vi "Heater Monitor.vi"() -> ()   [LabVIEW 2017]
uses:
  <vilib>/Utility/error.llb/Clear Errors.vi
  <instrlib>/tio-labview/TIO Library/Data Stream/TIO Data Stream Parse Description.vi
panel:
  in  "Voltage Max":dbl[unit] format="%#_4g"
  in  "Voltage Full Scale":dbl[unit] format="%#_4g"
  in  "Voltage":dbl[unit] format="%#_4g"
  in  "Manual":bool
  in  "Freq":dbl[unit] format="%#_4g"
  in  "Autostart":bool
  in  "Ki":dbl format="%#_4g"
  in  "Kp":dbl format="%#_4g"
  out "Resistance Measured":dbl[unit] format="%#_4g"
  in  "Save":bool
  in  "Calibrate R0":bool
  in  "Load":dbl[unit] format="%#_4g"
  in  "Heater Enable":bool
  out "Power Output":dbl[unit] format="%#_4f"
  in  "Power Max":dbl[unit] format="%#_4f"
  out "Temperature Measured":dbl[unit] format="%#_4g"
  in  "Temperature Set":dbl[unit] format="%#_4g"
  out "Kill":bool=TRUE
  in  "URL":refnum<visa-resource-name>="tcp://localhost"
  out "ID":string="Twinleaf VM4 R4"
  in  "Quit":bool
  in  "Duration":dbl[unit]=1000.0
  in  "Reset":bool
  out "Temperature":cluster{dbl, dbl, dbl[]}(graph)={407.109653, 0.002, []}
  # "Heater Monitor"
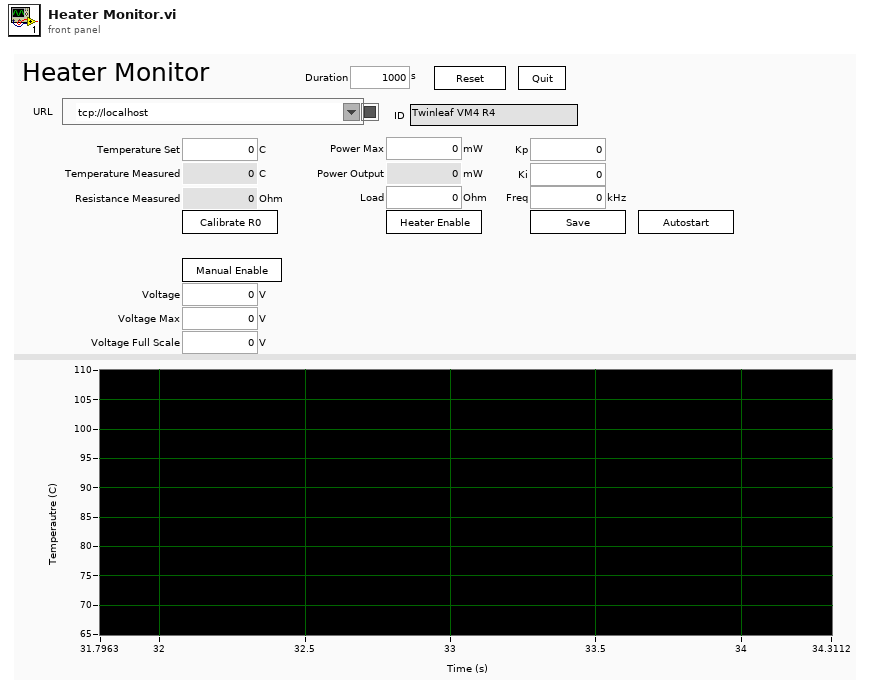
[diagram p1: front panel]
types:
  T1 = cluster{"Type":enum16{"TCP", "Serial"}, "Serial":refnum<visa-resource-name>, "TCP":refnum<k5>, "Timeout":u32}
  T2 = cluster{"Stream Description":cluster{"Stream ID":u16, "Data Type":u8, "Channels":u8, "Restart ID":u16, "Start timestamp (s)":dbl, "Sample counter":u64, "Period (s)":dbl, "Flags":u8, "Timestamp type":u8, "Name":string, "Last sample number":u64, "Last Restart ID":u16, "Version":u16, "Sample Size":u16}, "Sample #":u32, "Raw Data":string}
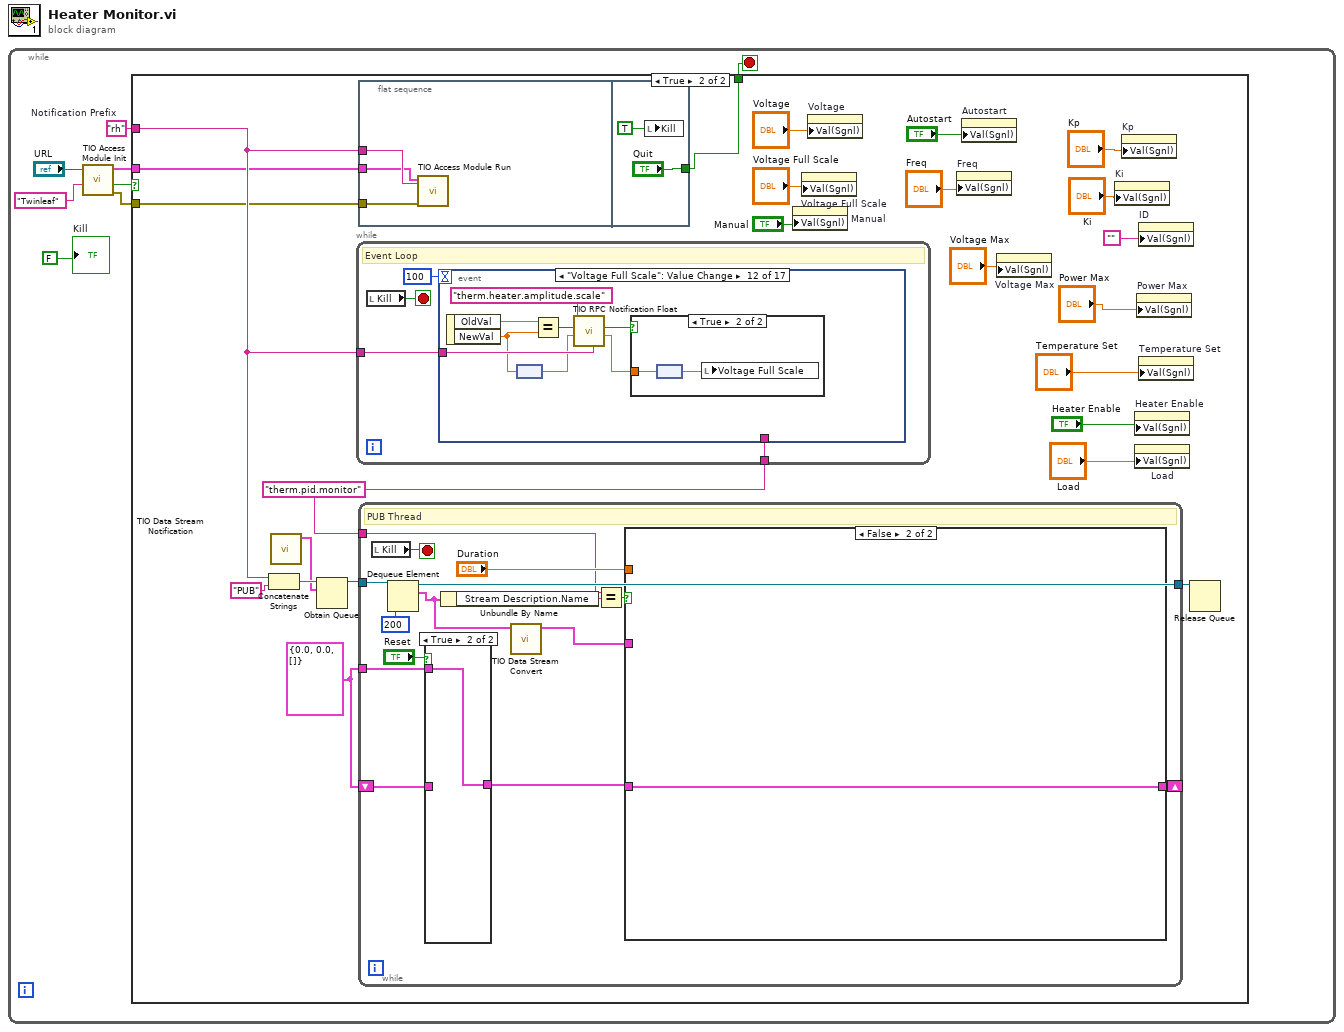
[diagram p0: block diagram]
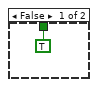
[diagram p2: hidden frame]
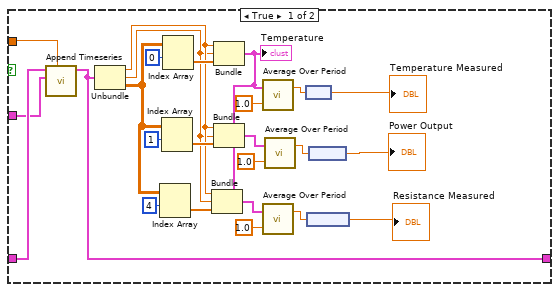
[diagram p4: hidden frame]
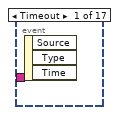
[diagram p5: hidden frame]
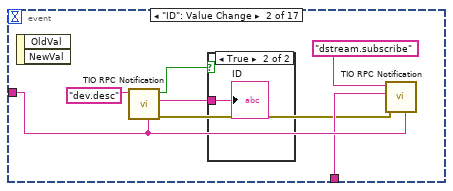
[diagram p6: hidden frame]
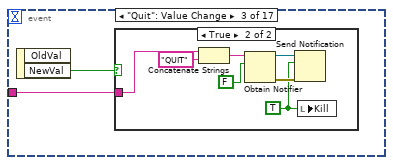
[diagram p8: hidden frame]
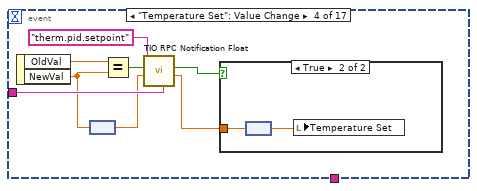
[diagram p10: hidden frame]
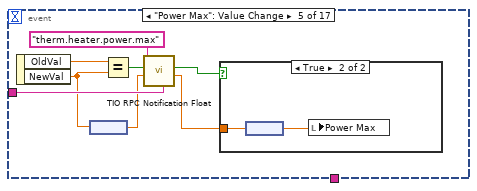
[diagram p12: hidden frame]
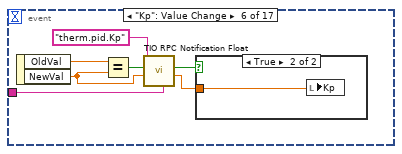
[diagram p14: hidden frame]
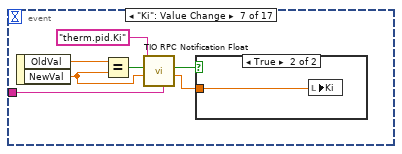
[diagram p16: hidden frame]
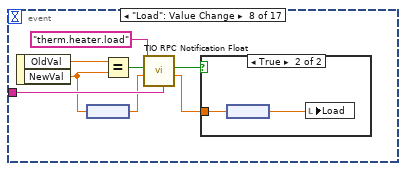
[diagram p18: hidden frame]
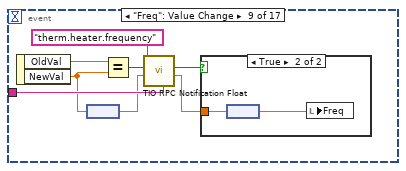
[diagram p20: hidden frame]
diagram:
  n1 = while {
    stop <- w1 stop-if-true
    w8 = "rh"  # Notification Prefix
    n2 = call <instrlib>:"TIO Access Module Init.vi"("ID"="Twinleaf", "URL"="URL") -> ("error out"=w5:errorcluster, "Connected"=w3:bool, "TS Connection"=w4:T1)  [unwired: 7 in]
    n3 = case shown="True" w3 {
      tunnel: w8 -> [_ w33]
      tunnel: w5 -> [_ w32]
      tunnel: w4 -> [_ w31]
      tunnel: [TRUE ("Quit") w14] -> w1
      frame False {
      }
      frame True {
        w15 = "therm.pid.monitor" ("Topic")
        w25 = cluster{dbl, dbl, dbl[][]} {0.0, 0.0, []} ("Waveform Timeseries")
        n4 = Concatenate Strings(w33, "PUB" ("name (unnamed)")) -> (w29:string)
        n5 = call <instrlib>:"TIO Data Stream Notification.vi"() -> ("Data Stream Notification"=w24:T2)  [unwired: 11 in]
        n6 = Obtain Queue(name (unnamed)=w29, element data type=w24) -> (queue out=w27:refnum<queue>)  [unwired: 3 in, 2 out]
        n7 = while {
          tunnel: w33 -> [w78]
          tunnel: w15 -> [w77]
          stop <- w80 stop-if-true
          # "Event Loop"
          n8 = local read "Kill"() -> (w80:bool)
          n9 = event shown="[11] \"Voltage Full Scale\": Value Change" {
            selector: _ -> [_ _ _ _ _ _ _ _ _ _ _ _ _ _ _ _ _]
            dyn-events: _ -> [_ _ _ _ _ _ _ _ _ _ _ _ _ _ _ _ _]
            timeout: 100 -> [_ _ _ _ _ _ _ _ _ _ _ _ _ _ _ _ _]
            tunnel: w78 -> [_ w83 w89 w105 w115 w124 w132 w141 w151 w161 w171 w181 w189 w199 w209 w215 w217]
            tunnel: w77 -> [_ w82 _ _ _ _ _ _ _ _ _ _ _ _ _ _ _]
            event Timeout {
              n10 = event-data() -> ()  [unwired: 1 in, 3 out]
            }
            event "ID": Value Change {
              n11 = event-data() -> ()  [unwired: 1 in, 2 out]
              n12 = call <instrlib>:"TIO RPC Notification.vi"("Notification Prefix"=w83, "Topic"="dev.desc") -> ("error out"=w81:errorcluster, "REP"=w86:string, "Response"=w85:bool)  [unwired: 6 in]
              n13 = case shown="True" w85 {
                tunnel: w86 -> [_ w88]
                frame False {
                }
                frame True {
                  "ID" <- w88
                }
              }
              n14 = call <instrlib>:"TIO RPC Notification.vi"("Notification Prefix"=w83, "error in (no error)"=w81, "Payload"=w82, "Topic"="dstream.subscribe") -> ()  [unwired: 4 in, 3 out]
            }
            event "Quit": Value Change {
              n15 = event-data() -> ("NewVal"=w90:bool)  [unwired: 1 in, 1 out]
              n16 = case shown="True" w90 {
                tunnel: w89 -> [_ w91]
                frame False {
                }
                frame True {
                  w92 = TRUE ("Kill")
                  n17 = Concatenate Strings(w91, "QUIT" ("name (unnamed)")) -> (w97:string)
                  n18 = Obtain Notifier(name (unnamed)=w97, notification data type=FALSE ("Connected")) -> (notifier out=w94:refnum<notifier>, error out=w95:errorcluster)  [unwired: 2 in, 1 out]
                  n19 = Send Notification(notification=w92, notifier=w94, error in (no error)=w95) -> ()  [unwired: 2 out]
                  n20 = local write "Kill"(w92) -> ()
                }
              }
            }
            event "Temperature Set": Value Change {
              n21 = event-data() -> ("OldVal"=w104:dbl[unit], "NewVal"=w98:dbl[unit])  [unwired: 1 in]
              n22 = node(w98) -> (w102:dbl)
              n23 = Equal?(x=w104, y=w98) -> (x = y?=w103:bool)
              n24 = call <instrlib>:"TIO RPC Notification Float.vi"("Notification"=w105, "Set value"=w102, "Read"=w103, "String"="therm.pid.setpoint") -> ("Get value (default if error)"=w100:sgl, "Response"=w101:bool)  [unwired: 4 in, 1 out]
              n25 = case shown="True" w101 {
                tunnel: w100 -> [_ w107]
                frame False {
                }
                frame True {
                  n26 = node(w107) -> (w106:sgl[unit])
                  n27 = local write "Temperature Set"(w106) -> ()
                }
              }
            }
            event "Power Max": Value Change {
              n28 = event-data() -> ("OldVal"=w114:dbl[unit], "NewVal"=w108:dbl[unit])  [unwired: 1 in]
              n29 = node(w108) -> (w112:dbl)
              n30 = Equal?(x=w114, y=w108) -> (x = y?=w113:bool)
              n31 = call <instrlib>:"TIO RPC Notification Float.vi"("Notification"=w115, "Set value"=w112, "Read"=w113, "String"="therm.heater.power.max") -> ("Get value (default if error)"=w110:sgl, "Response"=w111:bool)  [unwired: 4 in, 1 out]
              n32 = case shown="True" w111 {
                tunnel: w110 -> [_ w117]
                frame False {
                }
                frame True {
                  n33 = node(w117) -> (w116:sgl[unit])
                  n34 = local write "Power Max"(w116) -> ()
                }
              }
            }
            event "Kp": Value Change {
              n35 = event-data() -> ("OldVal"=w123:dbl, "NewVal"=w118:dbl)  [unwired: 1 in]
              n36 = Equal?(x=w123, y=w118) -> (x = y?=w122:bool)
              n37 = call <instrlib>:"TIO RPC Notification Float.vi"("Notification"=w124, "Set value"=w118, "Read"=w122, "String"="therm.pid.Kp") -> ("Get value (default if error)"=w120:sgl, "Response"=w121:bool)  [unwired: 4 in, 1 out]
              n38 = case shown="True" w121 {
                tunnel: w120 -> [_ w125]
                frame False {
                }
                frame True {
                  n39 = local write "Kp"(w125) -> ()
                }
              }
            }
            event "Ki": Value Change {
              n40 = event-data() -> ("OldVal"=w131:dbl, "NewVal"=w126:dbl)  [unwired: 1 in]
              n41 = Equal?(x=w131, y=w126) -> (x = y?=w130:bool)
              n42 = call <instrlib>:"TIO RPC Notification Float.vi"("Notification"=w132, "Set value"=w126, "Read"=w130, "String"="therm.pid.Ki") -> ("Get value (default if error)"=w128:sgl, "Response"=w129:bool)  [unwired: 4 in, 1 out]
              n43 = case shown="True" w129 {
                tunnel: w128 -> [_ w133]
                frame False {
                }
                frame True {
                  n44 = local write "Ki"(w133) -> ()
                }
              }
            }
            event "Load": Value Change {
              n45 = event-data() -> ("OldVal"=w140:dbl[unit], "NewVal"=w134:dbl[unit])  [unwired: 1 in]
              n46 = node(w134) -> (w138:dbl)
              n47 = Equal?(x=w140, y=w134) -> (x = y?=w139:bool)
              n48 = call <instrlib>:"TIO RPC Notification Float.vi"("Notification"=w141, "Set value"=w138, "Read"=w139, "String"="therm.heater.load") -> ("Get value (default if error)"=w136:sgl, "Response"=w137:bool)  [unwired: 4 in, 1 out]
              n49 = case shown="True" w137 {
                tunnel: w136 -> [_ w143]
                frame False {
                }
                frame True {
                  n50 = node(w143) -> (w142:sgl[unit])
                  n51 = local write "Load"(w142) -> ()
                }
              }
            }
            event "Freq": Value Change {
              n52 = event-data() -> ("OldVal"=w150:dbl[unit], "NewVal"=w144:dbl[unit])  [unwired: 1 in]
              n53 = node(w144) -> (w148:dbl)
              n54 = Equal?(x=w150, y=w144) -> (x = y?=w149:bool)
              n55 = call <instrlib>:"TIO RPC Notification Float.vi"("Notification"=w151, "Set value"=w148, "Read"=w149, "String"="therm.heater.frequency") -> ("Get value (default if error)"=w146:sgl, "Response"=w147:bool)  [unwired: 4 in, 1 out]
              n56 = case shown="True" w147 {
                tunnel: w146 -> [_ w153]
                frame False {
                }
                frame True {
                  n57 = node(w153) -> (w152:sgl[unit])
                  n58 = local write "Freq"(w152) -> ()
                }
              }
            }
            event "Voltage": Value Change {
              n59 = event-data() -> ("OldVal"=w160:dbl[unit], "NewVal"=w154:dbl[unit])  [unwired: 1 in]
              n60 = node(w154) -> (w158:dbl)
              n61 = Equal?(x=w160, y=w154) -> (x = y?=w159:bool)
              n62 = call <instrlib>:"TIO RPC Notification Float.vi"("Notification"=w161, "Set value"=w158, "Read"=w159, "String"="therm.heater.amplitude") -> ("Get value (default if error)"=w156:sgl, "Response"=w157:bool)  [unwired: 4 in, 1 out]
              n63 = case shown="True" w157 {
                tunnel: w156 -> [_ w163]
                frame False {
                }
                frame True {
                  n64 = node(w163) -> (w162:sgl[unit])
                  n65 = local write "Voltage"(w162) -> ()
                }
              }
            }
            event "Voltage Max": Value Change {
              n66 = event-data() -> ("OldVal"=w170:dbl[unit], "NewVal"=w164:dbl[unit])  [unwired: 1 in]
              n67 = node(w164) -> (w168:dbl)
              n68 = Equal?(x=w170, y=w164) -> (x = y?=w169:bool)
              n69 = call <instrlib>:"TIO RPC Notification Float.vi"("Notification"=w171, "Set value"=w168, "Read"=w169, "String"="therm.heater.amplitude.max") -> ("Get value (default if error)"=w166:sgl, "Response"=w167:bool)  [unwired: 4 in, 1 out]
              n70 = case shown="True" w167 {
                tunnel: w166 -> [_ w173]
                frame False {
                }
                frame True {
                  n71 = node(w173) -> (w172:sgl[unit])
                  n72 = local write "Voltage Max"(w172) -> ()
                }
              }
            }
            event "Voltage Full Scale": Value Change {
              n73 = event-data() -> ("OldVal"=w180:dbl[unit], "NewVal"=w174:dbl[unit])  [unwired: 1 in]
              n74 = node(w174) -> (w178:dbl)
              n75 = Equal?(x=w180, y=w174) -> (x = y?=w179:bool)
              n76 = call <instrlib>:"TIO RPC Notification Float.vi"("Notification"=w181, "Set value"=w178, "Read"=w179, "String"="therm.heater.amplitude.scale") -> ("Get value (default if error)"=w176:sgl, "Response"=w177:bool)  [unwired: 4 in, 1 out]
              n77 = case shown="True" w177 {
                tunnel: w176 -> [_ w183]
                frame False {
                }
                frame True {
                  n78 = node(w183) -> (w182:sgl[unit])
                  n79 = local write "Voltage Full Scale"(w182) -> ()
                }
              }
            }
            event "Heater Enable": Value Change {
              n80 = event-data() -> ("OldVal"=w191:bool, "NewVal"=w184:bool)  [unwired: 1 in]
              n81 = Equal?(x=w191, y=w184) -> (x = y?=w188:bool)
              n82 = Boolean To (0,1)(Boolean=w184) -> (0, 1=w190:i16)
              n83 = call <instrlib>:"TIO RPC Notification U8.vi"("Notification Prefix"=w189, "U8"=w190, "Read"=w188, "String"="therm.pid.enable") -> ("U8"=w185:u8, "Response"=w186:bool)  [unwired: 4 in, 1 out]
              n84 = case shown="True" w186 {
                tunnel: w185 -> [_ w193]
                frame False {
                }
                frame True {
                  n85 = Greater Than 0?(x=w193) -> (x > 0?=w192:bool)
                  n86 = local write "Heater Enable"(w192) -> ()
                }
              }
            }
            event "Autostart": Value Change {
              n87 = event-data() -> ("OldVal"=w201:bool, "NewVal"=w194:bool)  [unwired: 1 in]
              n88 = Equal?(x=w201, y=w194) -> (x = y?=w198:bool)
              n89 = Boolean To (0,1)(Boolean=w194) -> (0, 1=w200:i16)
              n90 = call <instrlib>:"TIO RPC Notification U8.vi"("Notification Prefix"=w199, "U8"=w200, "Read"=w198, "String"="autostart") -> ("U8"=w195:u8, "Response"=w196:bool)  [unwired: 4 in, 1 out]
              n91 = case shown="True" w196 {
                tunnel: w195 -> [_ w203]
                frame False {
                }
                frame True {
                  n92 = Greater Than 0?(x=w203) -> (x > 0?=w202:bool)
                  n93 = local write "Autostart"(w202) -> ()
                }
              }
            }
            event "Manual": Value Change {
              n94 = event-data() -> ("OldVal"=w211:bool, "NewVal"=w204:bool)  [unwired: 1 in]
              n95 = Equal?(x=w211, y=w204) -> (x = y?=w208:bool)
              n96 = Boolean To (0,1)(Boolean=w204) -> (0, 1=w210:i16)
              n97 = call <instrlib>:"TIO RPC Notification U8.vi"("Notification Prefix"=w209, "U8"=w210, "Read"=w208, "String"="therm.pid.manual") -> ("U8"=w205:u8, "Response"=w206:bool)  [unwired: 4 in, 1 out]
              n98 = case shown="True" w206 {
                tunnel: w205 -> [_ w213]
                frame False {
                }
                frame True {
                  n99 = Greater Than 0?(x=w213) -> (x > 0?=w212:bool)
                  n100 = local write "Manual"(w212) -> ()
                }
              }
            }
            event "Calibrate R0": Value Change {
              n101 = event-data() -> ()  [unwired: 1 in, 2 out]
              n102 = call <instrlib>:"TIO RPC Notification.vi"("Notification Prefix"=w215, "Topic"="therm.R0.capture" ("String")) -> ()  [unwired: 6 in, 3 out]
            }
            event "Save": Value Change {
              n103 = event-data() -> ()  [unwired: 1 in, 2 out]
              n104 = call <instrlib>:"TIO RPC Notification.vi"("Notification Prefix"=w217, "Topic"="conf.save" ("String")) -> ()  [unwired: 6 in, 3 out]
            }
          }
        }
        n105 = flat-sequence {
          tunnel: w33 -> [w220]
          tunnel: w32 -> [w219]
          tunnel: w31 -> [w218]
          tunnel: ["Quit"] -> _
          tunnel: ["Quit"] -> w14
          frame #0 {
            n106 = call <instrlib>:"TIO Access Module Run.vi"("Notification Prefix"=w220, "error in (no error)"=w219, "TS Connection"=w218) -> ()  [unwired: 9 in]
          }
          frame #1 {
            n107 = local write "Kill"(TRUE ("Kill")) -> ()
          }
        }
        n108 = while {
          tunnel: w27 -> [w46]
          shift-right: [w45] -> _
          shift-left: w25 -> [w43]
          tunnel: w25 -> [w42]
          tunnel: [w39] -> w26
          tunnel: w15 -> [w34]
          stop <- w47 stop-if-true
          # "PUB Thread"
          n109 = local read "Kill"() -> (w47:bool)
          n110 = Dequeue Element(queue=w46, timeout in ms (-1)=200) -> (queue out=w39:refnum<queue>, element=w37:T2)  [unwired: 1 in, 2 out]
          n111 = case shown="True" "Reset" {
            tunnel: w43 -> [w49 _]
            tunnel: [w49 w50] -> w41
            tunnel: w42 -> [_ w50]
            frame False {
            }
            frame True {
            }
          }
          n112 = Unbundle By Name(w37) -> ("Stream Description.Name"=w36:string)
          n113 = call <instrlib>:"TIO Data Stream Convert.vi"("Data Stream Notification"=w37) -> ("Waveform"=w38:cluster{dbl, dbl, dbl[][]})  [unwired: 10 in]
          n114 = Equal?(x=w34, y=w36) -> (x = y?=w35:bool)
          n115 = case shown="False" w35 {
            tunnel: "Duration" -> [w75 _]
            tunnel: [w73 w76] -> w45
            tunnel: w41 -> [w72 w76]
            tunnel: w38 -> [w70 _]
            frame True {
              n116 = call <instrlib>:"Append Timeseries.vi"("Duration"=w75, "Waveform New"=w70, "Waveform History"=w72) -> ("Waveform Timeseries"=w73:cluster{dbl, dbl, dbl[][]})  [unwired: 8 in]
              n117 = Unbundle(w73) -> (w53:dbl, w52:dbl, w55:dbl[][])
              n118 = Index Array(array=w55, index (row)=4 ("disabled index (col)")) -> (element=w57:dbl[])  [unwired: 1 in]
              n119 = Index Array(array=w55, index (row)=1 ("disabled index (col)")) -> (element=w65:dbl[])  [unwired: 1 in]
              n120 = Index Array(array=w55, index (row)=0 ("disabled index (col)")) -> (element=w71:dbl[])  [unwired: 1 in]
              n121 = Bundle(w53, w52, w71) -> (w54:cluster{dbl, dbl, dbl[]})  [unwired: 1 in]
              "Temperature" <- w54
              n122 = Bundle(cluster=w54, w53, w52, w57) -> (w59:cluster{dbl, dbl, dbl[]})
              n123 = Bundle(cluster=w54, w53, w52, w65) -> (w63:cluster{dbl, dbl, dbl[]})
              n124 = call <instrlib>:"Average Over Period.vi"("Period"=dbl[unit] 1.0, "Cluster"=w54) -> ("Average"=w68:dbl)  [unwired: 1 in]
              n125 = call <instrlib>:"Average Over Period.vi"("Period"=dbl[unit] 1.0, "Cluster"=w59) -> ("Average"=w60:dbl)  [unwired: 1 in]
              n126 = call <instrlib>:"Average Over Period.vi"("Period"=dbl[unit] 1.0, "Cluster"=w63) -> ("Average"=w62:dbl)  [unwired: 1 in]
              n127 = node(w68) -> (→"Temperature Measured":dbl[unit])
              n128 = node(w60) -> (→"Resistance Measured":dbl[unit])
              n129 = node(w62) -> (→"Power Output":dbl[unit])
            }
            frame False {
            }
          }
        }
        n130 = property on="Manual" class="Bool (strict)"("Val(Sgnl)"="Manual") -> ()  [unwired: 2 in, 2 out]
        n131 = property on="Voltage Full Scale" class="DigNum (strict)"("Val(Sgnl)"="Voltage Full Scale") -> ()  [unwired: 2 in, 2 out]
        n132 = property on="Voltage" class="DigNum (strict)"("Val(Sgnl)"="Voltage") -> ()  [unwired: 2 in, 2 out]
        n133 = property on="Freq" class="DigNum (strict)"("Val(Sgnl)"="Freq") -> ()  [unwired: 2 in, 2 out]
        n134 = property on="Autostart" class="Bool (strict)"("Val(Sgnl)"="Autostart") -> ()  [unwired: 2 in, 2 out]
        n135 = property on="Voltage Max" class="DigNum (strict)"("Val(Sgnl)"="Voltage Max") -> ()  [unwired: 2 in, 2 out]
        n136 = property on="Ki" class="DigNum (strict)"("Val(Sgnl)"="Ki") -> ()  [unwired: 2 in, 2 out]
        n137 = property on="Kp" class="DigNum (strict)"("Val(Sgnl)"="Kp") -> ()  [unwired: 2 in, 2 out]
        n138 = property on="Heater Enable" class="Bool (strict)"("Val(Sgnl)"="Heater Enable") -> ()  [unwired: 2 in, 2 out]
        n139 = property on="Load" class="DigNum (strict)"("Val(Sgnl)"="Load") -> ()  [unwired: 2 in, 2 out]
        n140 = property on="Power Max" class="DigNum (strict)"("Val(Sgnl)"="Power Max") -> ()  [unwired: 2 in, 2 out]
        n141 = property on="ID" class="Str"("Val(Sgnl)"="") -> ()  [unwired: 2 in, 2 out]
        n142 = property on="Temperature Set" class="DigNum (strict)"("Val(Sgnl)"="Temperature Set") -> ()  [unwired: 2 in, 2 out]
        n143 = Release Queue(queue=w26) -> ()  [unwired: 2 in, 3 out]
      }
    }
    "Kill" <- FALSE ("Kill")
  }
